vi "ARB SEL TEST MODEL.vi"(4 "LTE BW (MHz)":dbl, 6 "Test Model":u16(ring) items=["E-TM1-1", "E-TM2", "E-TM3-1", "E-TM3-2", "E-TM3-3"], 7 "Timeout":u32=3000, 8 "error in":errorcluster {"code" format="%.0x"}, 11 "Session In":refnum<visa-resource-name>="TCPIP0::A-N5182B-052670::inst0::INSTR") -> (0 "error out":errorcluster {"code" format="%.0x"}, 3 "Session Out":refnum<visa-resource-name>)   [LabVIEW 2018]
panel:
  in  "Bandwidth (MHz)":u16(ring) items=["1.4", "3", "5", "10", "15", "20"]
  out "output string":string
  out "READ WFM1":string
  # "File Names\n\nE-TM1_1_10(50RB).wfm\nE-TM1_1_15(75RB).wfm\nE-TM1_1_1P4(6RB).wfm\nE-TM1_1_20(100RB).wfm\nE-TM1_1_3(15RB).wfm\nE-TM1_1_5(25RB).wfm\nE-TM1_2_10(50RB).wfm\nE-TM1_2_15(75RB).wfm\nE-TM1_2_1P4(6RB).wfm\nE-TM1_2_20(100RB).wfm\nE-TM1_2_3(15RB).wfm\nE-TM1_2_5(25RB).wfm\nE-TM2_0_10(50RB).wfm\nE-TM2_0_15(75RB).wfm\nE-TM2_0_1P4(6RB).wfm\nE-TM2_0_20(100RB).wfm\nE-TM2_0_5(25RB).wfm\nE-TM2_2_3(15RB).wfm\nE-TM3_1_10(50RB).wfm\nE-TM3_1_15(75RB).wfm\nE-TM3_1_1P4(6RB).wfm\nE-TM3_1_20(100RB).wfm\nE-TM3_1_3(15RB).wfm\nE-TM3_1_5(25RB).wfm\nE-TM3_2_10(50RB).wfm\nE-TM3_2_15(75RB).wfm\nE-TM3_2_1P4(6RB).wfm\nE-TM3_2_20(100RB).wfm\nE-TM3_2_3(15RB).wfm\nE-TM3_2_5(25RB).wfm\nE-TM3_3_10(50RB).wfm\nE-TM3_3_15(75RB).wfm\nE-TM3_3_1P4(6RB).wfm\nE-TM3_3_20(100RB).wfm\nE-TM3_3_3(15RB).wfm\nE-TM3_3_5(25RB).wfm"
  # "N5182B : Use This vi to load the waveforms into ARB"
  # "Filenames were created by Rage and must be correct"
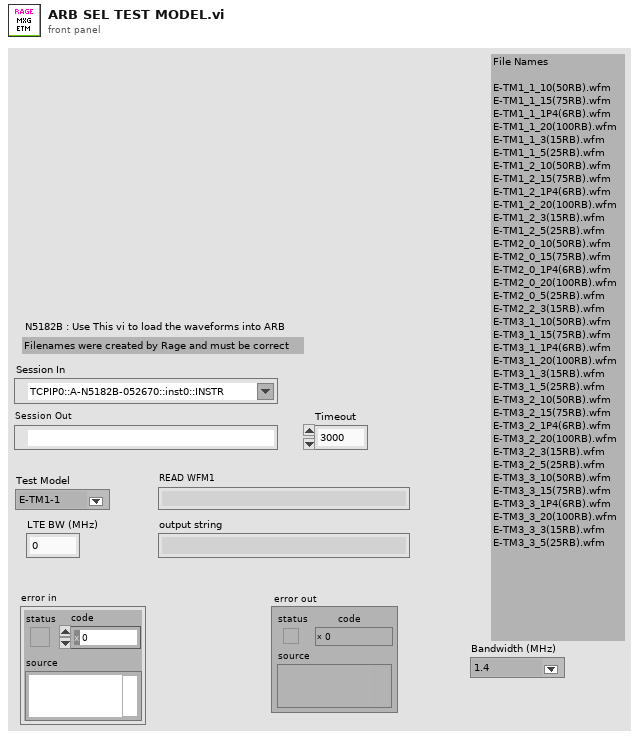
[diagram p1: front panel]
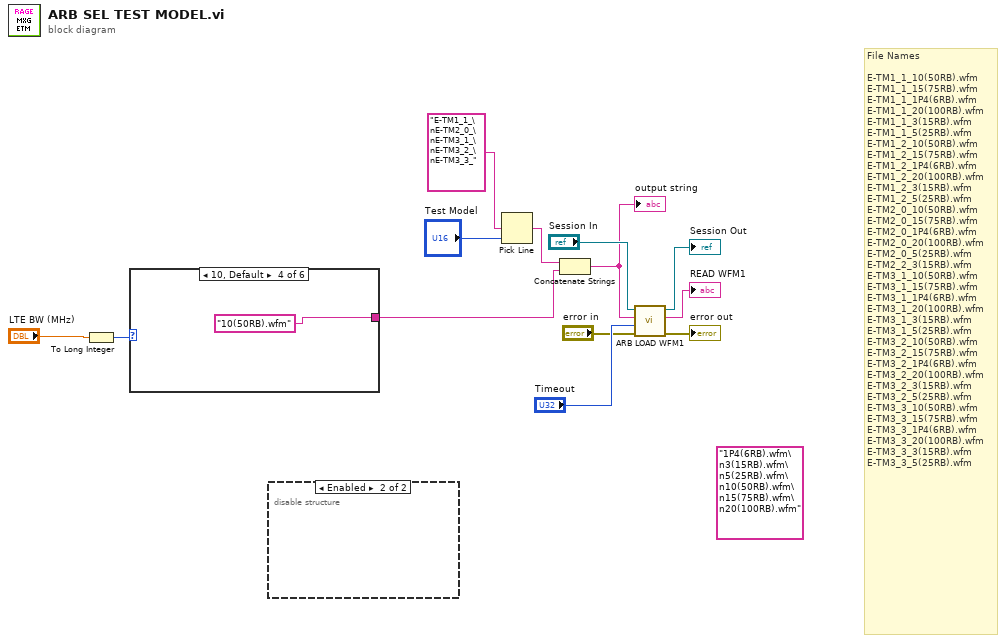
[diagram p0: block diagram]
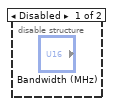
[diagram p2: hidden frame]
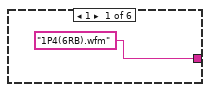
[diagram p3: hidden frame]
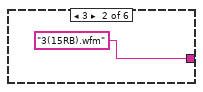
[diagram p4: hidden frame]
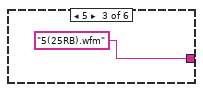
[diagram p5: hidden frame]
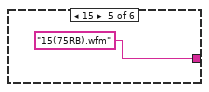
[diagram p6: hidden frame]
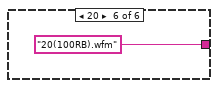
[diagram p7: hidden frame]
diagram:
  (unwired) "1P4(6RB).wfm\n3(15RB).wfm\n5(25RB).wfm\n10(50RB).wfm\n15(75RB).wfm\n20(100RB).wfm" ("WRITE WFM1")
  # "File Names\n\nE-TM1_1_10(50RB).wfm\nE-TM1_1_15(75RB).wfm\nE-TM1_1_1P4(6RB).wfm\nE-TM1_1_20(100RB).wfm\nE-TM1_1_3(15RB).wfm\nE-TM1_1_5(25RB).wfm\nE-TM1_2_10(50RB).wfm\nE-TM1_2_15(75RB).wfm\nE-TM1_2_1P4(6RB).wfm\nE-TM1_2_20(100RB).wfm\nE-TM1_2_3(15RB).wfm\nE-TM1_2_5(25RB).wfm\nE-TM2_0_10(50RB).wfm\nE-TM2_0_15(75RB).wfm\nE-TM2_0_1P4(6RB).wfm\nE-TM2_0_20(100RB).wfm\nE-TM2_0_5(25RB).wfm\nE-TM2_2_3(15RB).wfm\nE-TM3_1_10(50RB).wfm\nE-TM3_1_15(75RB).wfm\nE-TM3_1_1P4(6RB).wfm\nE-TM3_1_20(100RB).wfm\nE-TM3_1_3(15RB).wfm\nE-TM3_1_5(25RB).wfm\nE-TM3_2_10(50RB).wfm\nE-TM3_2_15(75RB).wfm\nE-TM3_2_1P4(6RB).wfm\nE-TM3_2_20(100RB).wfm\nE-TM3_2_3(15RB).wfm\nE-TM3_2_5(25RB).wfm\nE-TM3_3_10(50RB).wfm\nE-TM3_3_15(75RB).wfm\nE-TM3_3_1P4(6RB).wfm\nE-TM3_3_20(100RB).wfm\nE-TM3_3_3(15RB).wfm\nE-TM3_3_5(25RB).wfm"
  n1 = To Long Integer(number="LTE BW (MHz)") -> (32bit integer=w2:i32)
  n2 = case shown="10, Default" w2 {
    tunnel: ["1P4(6RB).wfm" ("WRITE WFM1") "3(15RB).wfm" ("WRITE WFM1") "5(25RB).wfm" ("WRITE WFM1") "10(50RB).wfm" ("WRITE WFM1") "15(75RB).wfm" ("WRITE WFM1") "20(100RB).wfm" ("WRITE WFM1")] -> w3
    frame 1 {
    }
    frame 3 {
    }
    frame 5 {
    }
    frame 10, Default {
    }
    frame 15 {
    }
    frame 20 {
    }
  }
  n3 = disable-structure shown="Enabled" {
    frame Disabled {
    }
    frame Enabled {
    }
  }
  n4 = Pick Line(multi-line string="E-TM1_1_\nE-TM2_0_\nE-TM3_1_\nE-TM3_2_\nE-TM3_3_" ("WRITE WFM1"), line index="Test Model") -> (output string=w9:string)  [unwired: 1 in]
  n5 = Concatenate Strings(w9, w3) -> (w8:string)
  "output string" <- w8
  n6 = call "ARB LOAD WFM1.vi"("error in"="error in", "Timeout"="Timeout", "WRITE WFM1"=w8, "Session In"="Session In") -> ("error out"=→"error out":errorcluster, "READ WFM1"=→"READ WFM1":string, "Session Out"=→"Session Out":refnum<visa-resource-name>)  [unwired: 5 in]
